vi "GetCommandsFromFile.vi"(8 "error in":errorcluster, 11 "Path":path) -> (0 "error out":errorcluster, 1 "Parameters_PositionProfile":dbl[](array[numeric]), 4 "Parameters_Reference":dbl[](array[numeric]))   [LabVIEW 2017]
uses:
  Utilities/WordManipulationLibrary.lvlib
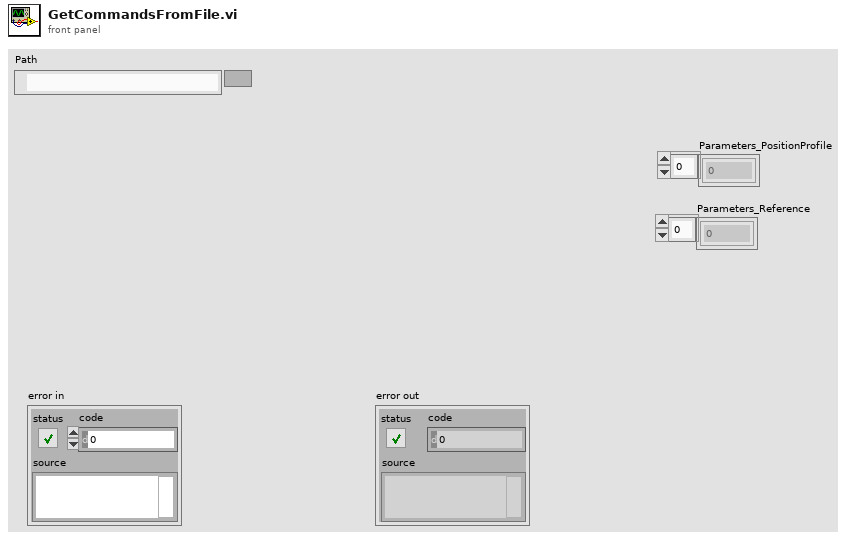
[diagram p1: front panel]
types:
  T1 = enum16{"Shutdown", "Switch On", "Disable Voltage", "Quick Stop", "Disable Op", "Enable Op", "Fault Reset", "Error"}
  T2 = enum16{"Shutdown", "Switch On", "Disable Voltage", "Quick Stop", "Disable Op", "Enable Op", "Fault Reset", "Error"}[]
  T3 = enum16{"Reserved", "Profile Position Mode", "Velocity Mode", "Profile Velocity Mode", "Profile Torque Mode", "Reserved 2", "Reference Mode", "Interpolated Position Mode", "Skip"}[]
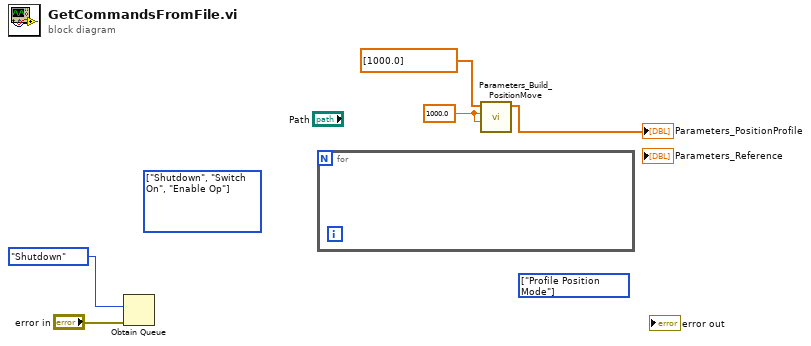
[diagram p0: block diagram]
diagram:
  (unwired) T2 [enum."Shutdown", enum."Switch On", enum."Enable Op"] items=["Shutdown", "Switch On", "Disable Voltage", "Quick Stop", "Disable Op", "Enable Op", "Fault Reset", "Error"] ("Device Control")
  w3 = 1000.0 ("Velocity")
  (unwired) T3 [enum."Profile Position Mode"] items=["Reserved", "Profile Position Mode", "Velocity Mode", "Profile Velocity Mode", "Profile Torque Mode", "Reserved 2", "Reference Mode", "Interpolated Position Mode", "Skip"] ("Command Array")
  n1 = Obtain Queue(element data type=T1."Shutdown" ("Device Control Command"), error in (no error)="error in") -> ()  [unwired: 3 in, 3 out]
  n2 = for {
  }
  n3 = call "Parameters_Build_PositionMove.vi"("Acceleration"=w3, "Velocity"=w3, "Positions"=dbl[] [1000.0]) -> ("Parameters"=→"Parameters_PositionProfile":dbl[])  [unwired: 8 in]
